vi "FPGA 5 Wire xVDT Sim.vi"() -> ()   [LabVIEW 2010]
uses:
  <vilib>/eio/EIONode/EIONode.xnode
  <vilib>/rvi/eio/nirviEIOImplementation/nirviEIOImplementation.xnode
  <vilib>/rvi/eio/common/nirviEmuClasses.ctl
  <vilib>/rvi/eio/common/nirviEmuTemplateMethod_noerrors.vi
panel:
  in  "Scaling Factor":fxp<+/-,19,5>
  in  "Scaling Factor 2":fxp<+/-,19,5>
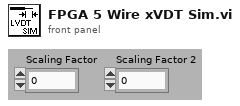
[diagram p1: front panel]
types:
  T1 = typedef "nirviEmuClasses.ctl" = enum16{"IO Read", "IO Write", "Method", "Property Read", "Property Write"}
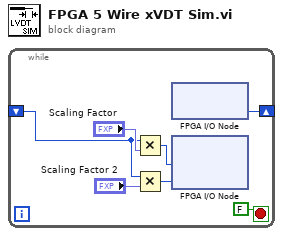
[diagram p0: block diagram]
diagram:
  n1 = while {
    shift-right: [w4] -> _
    shift-left: _ -> [w3]
    stop <- FALSE stop-if-true
    n2 = Multiply(x=w3, y="Scaling Factor") -> (x*y=w2:i16)
    n3 = Multiply(x=w3, y="Scaling Factor 2") -> (x*y=w1:i16)
    n4 = xnode "FPGA I/O Node"() -> ("AI0"=w4:i16)  [unwired: 1 in, 1 out]
    n5 = xnode "FPGA I/O Node"("AO0"=w2, "AO1"=w1) -> ()  [unwired: 2 in, 2 out]
  }
